vi "Close.vi"(8 "error in (no error)":errorcluster, 10 "Sequence Context":refnum<k7>, 11 "TestExec in":refnum<class "TestExec.lvclass">) -> (0 "error out":errorcluster, 3 "TestExec out":refnum<class "TestExec.lvclass">)   [LabVIEW 2019, in "Sequence Main.lvlib" / "TestExec.lvclass"]
uses:
  TestExec.lvclass
  TestExec.lvclass/TestExec.ctl
  <vilib>/addons/TestStand/_TSUtility.llb/TestStand - Set Property Value (Boolean).vi
  Abstract UUT/Abstract UUT.lvclass
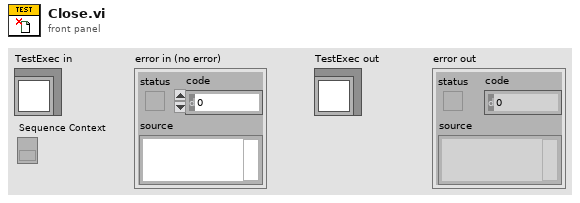
[diagram p1: front panel]
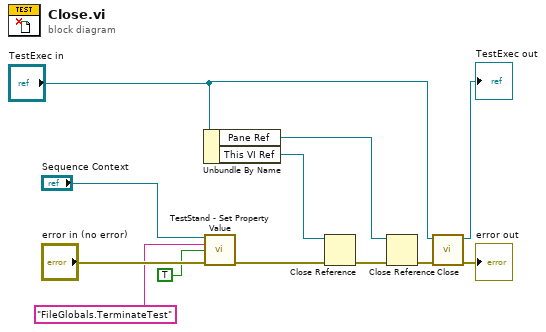
[diagram p0: block diagram]
diagram:
  n1 = Unbundle By Name("TestExec in") -> ("Pane Ref"=w10:refnum<vi>, "This VI Ref"=w8:refnum<vi>)
  n2 = call-poly <vilib>:"TestStand - Set Property Value.vi"("Sequence Context In"="Sequence Context", "Lookup String"="FileGlobals.TerminateTest", "New Value"=TRUE, "error in (no error)"="error in (no error)") -> ("error out"=w4:errorcluster)  [unwired: 10 in, 1 out]
  n3 = Close Reference(reference=w8, error in (no error)=w4) -> (error out=w9:errorcluster)
  n4 = Close Reference(reference=w10, error in (no error)=w9) -> (error out=w7:errorcluster)
  n5 = call-parent "Close.vi"("error in (no error)"=w7, "Abstract UUT in"="TestExec in") -> ("error out"=→"error out":errorcluster, "Abstract UUT out"=→"TestExec out":refnum<class "TestExec.lvclass">)  [unwired: 8 in]
